vi "Get EPICS server attributes.vi"(8 "error in (no error)":errorcluster, 11 "EPICS server ref in":refnum<data-value>) -> (0 "error out":errorcluster, 2 "EPICS server attributes":T2(array[cluster]), 3 "EPICS server ref out":refnum<data-value>)   [LabVIEW 2011]
uses:
  <vilib>/variable/tagger/epicsserver/API/internal/EPICSServerClass/EPICSServer.lvclass
  <vilib>/lvdsc/process/internal/data type.ctl
  <vilib>/variable/tagger/epicsserver/API/internal/List PVs (By Ref).vi
  <vilib>/variable/tagger/epicsserver/API/NI_EPICS_Server.lvlib
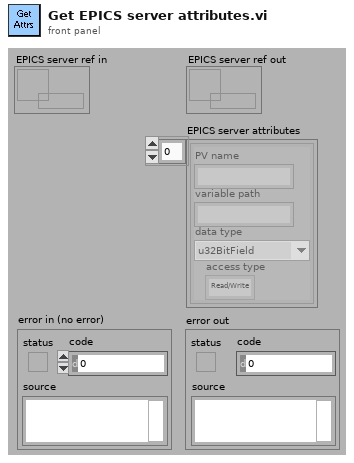
[diagram p1: front panel]
types:
  T1 = typedef "data type.ctl" = enum32{"u32BitField", "bool", "double", "string", "int8", "uint8", "int16", "uint16", "int32", "uint32", "int64", "uint64", "single", "double waveform", "int16 waveform", "array of boolean", "array of int8", "array of uint8", "array of int16", "array of uint16", "array of int32", "array of uint32", "array of int64", "array of uint64", "array of single", "array of double", "array of double waveform", "array of int16 waveform", "array of string", "variant", "timestamp", "fixed point", "custom"}
  T2 = cluster{"PV name":string, "variable path":string, "data type":T1, "access type":enum16{"Read/Write", "Read Only"}}[]
  T3 = cluster{"PV name":string, "variable path":string, "data type":T1, "access type":enum16{"Read/Write", "Read Only"}}
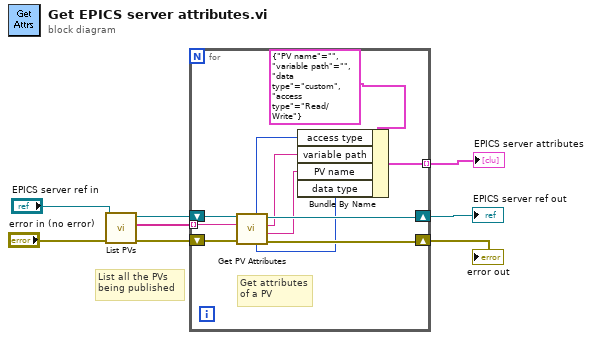
[diagram p0: block diagram]
diagram:
  # "List all the PVs\nbeing published"
  n1 = call-poly <vilib>:"List PVs.vi"("error in (no error)"="error in (no error)", "EPICS Server ref in"="EPICS server ref in") -> ("error out"=w6:errorcluster, "PVs"=w7:string[], "EPICS Server ref out"=w8:refnum<data-value>)  [unwired: 7 in]
  n2 = for {
    shift-right: [w18] -> w3
    shift-left: w8 -> [w19]
    tunnel: w7 -> [w17] mode=indexing
    shift-right: [w15] -> w2
    shift-left: w6 -> [w16]
    tunnel: [w10] -> w1 mode=indexing
    # "Get attributes\nof a PV"
    n3 = call <vilib>:"Get PV Attributes.vi"("error in (no error)"=w16, "PV name or variable path"=w17, "EPICS Server ref in"=w19) -> ("error out"=w15:errorcluster, "PV name"=w12:string, "variable path"=w13:string, "EPICS Server ref out"=w18:refnum<data-value>, "data type"=w11:u16, "access type"=w14:u16)  [unwired: 2 in, 1 out]
    n4 = Bundle By Name(cluster=T3 {"PV name"="", "variable path"="", "data type"=enum."custom", "access type"=enum."Read/Write"} ("element"), "access type"=w14, "variable path"=w13, "PV name"=w12, "data type"=w11) -> (w10:T3)
  }
  "EPICS server ref out" <- w3
  "error out" <- w2
  "EPICS server attributes" <- w1
